vi "Warnings.vi"() -> ()   [LabVIEW 2014]
doc: "This VI takes current temp, minimum temp and max temp and then comapres the data to issue either no warning, a freeze warning, or a heatstroke warning. \n\nCreated by Lee Martin\nSept 14-15, 2016"
panel:
  out "Warning?":bool
  out "Warning Text":string
  in  "Min Temp":dbl
  in  "Max Temp":dbl
  in  "Current Temp":dbl
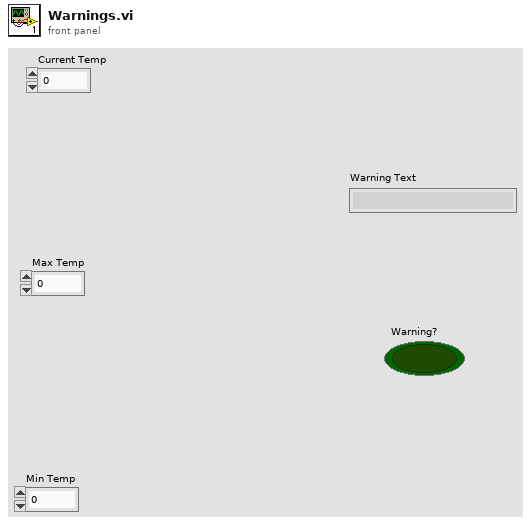
[diagram p1: front panel]
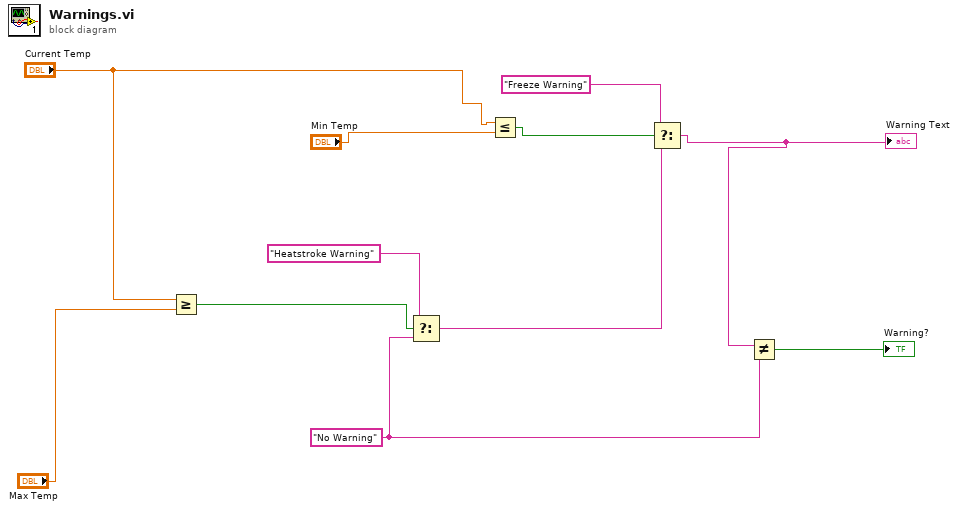
[diagram p0: block diagram]
diagram:
  w3 = "No Warning"
  n1 = Greater Or Equal?(x="Current Temp", y="Max Temp") -> (x >= y?=w6:bool)
  n2 = Select(t="Heatstroke Warning", s=w6, f=w3) -> (s? t:f=w2:string)
  n3 = Less Or Equal?(x="Current Temp", y="Min Temp") -> (x <= y?=w8:bool)
  n4 = Select(t="Freeze Warning", s=w8, f=w2) -> (s? t:f=w7:string)
  "Warning Text" <- w7
  n5 = Not Equal?(x=w7, y=w3) -> (x != y?=→"Warning?":bool)
